vi "capture.vi"(8 "error in (no error)":errorcluster, 11 "object in":refnum<class "Piece.lvclass">) -> (0 "error out":errorcluster, 3 "object out":refnum<class "Piece.lvclass">)   [LabVIEW 2020, in "Piece.lvclass"]
uses:
  Piece.lvclass
  Piece.lvclass/Piece.ctl
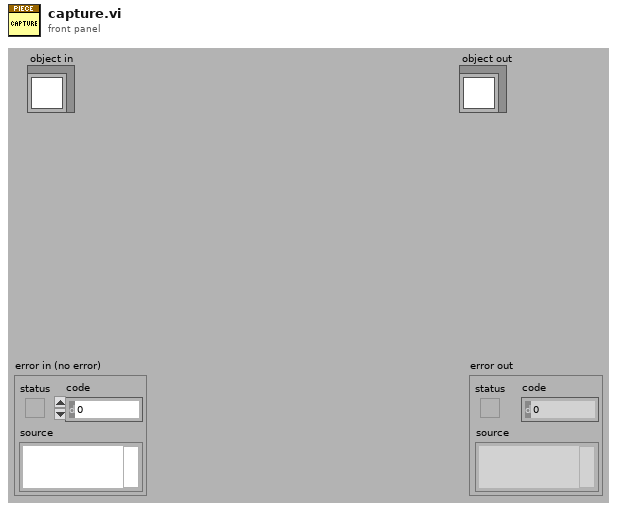
[diagram p1: front panel]
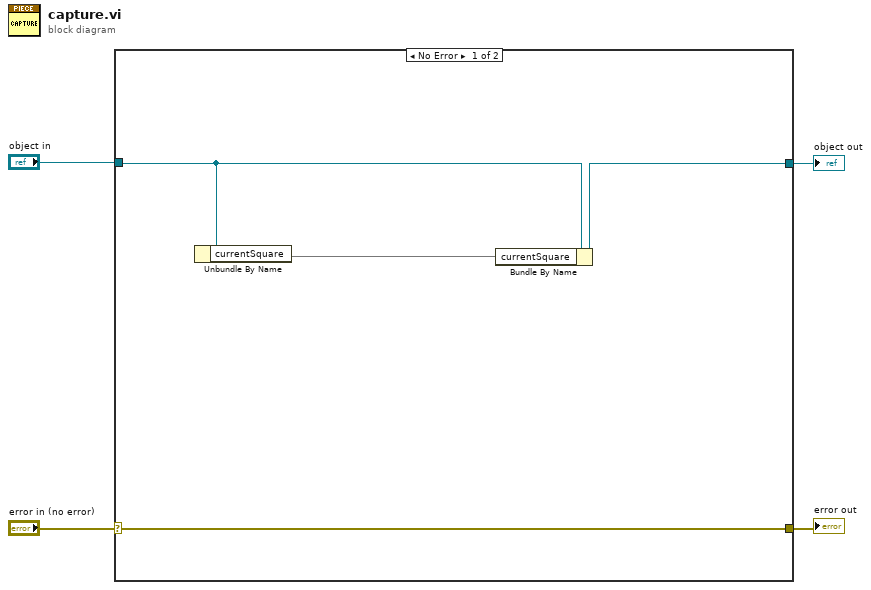
[diagram p0: block diagram]
diagram:
  n1 = case shown="No Error" "error in (no error)" {
    selector: "error in (no error)" -> [w7 w10]
    tunnel: [w7 w10] -> w3
    tunnel: [w5 w9] -> w1
    tunnel: "object in" -> [w6 w9]
    frame No Error {
      n2 = Unbundle By Name(w6) -> ("currentSquare"=w8:map{string, i32})
      n3 = Bundle By Name(cluster=w6, "currentSquare"=w8) -> (w5:refnum<class "Piece.lvclass">)
    }
    frame Error {
    }
  }
  "error out" <- w3
  "object out" <- w1
